vi "Webcam - Clamp Edges.vi"(0 "Image In":T1, 5 "Search Area Left":i32, 7 "Search Area Top":i32, 9 "Search Area Right":i32, 11 "Search Area Bottom":i32, 12 "Settings":T2={"Contrast"=100, "Filter width"=100, "Steepness"=2, "Subsampling Ratio"=1, "Show Search Area"=FALSE, "Show Search Lines"=FALSE, "Show Edges Found"=FALSE, "Show Result"=FALSE}) -> (4 "Image Out":T1, 6 "Left":sgl, 8 "Bottom":sgl, 10 "Right":sgl, 15 "Top":sgl)   [LabVIEW 2011]
uses:
  <vilib>/vision/Image Controls.llb/IMAQ Image.ctl
  <vilib>/vision/NI_Vision_Development_Module.lvlib
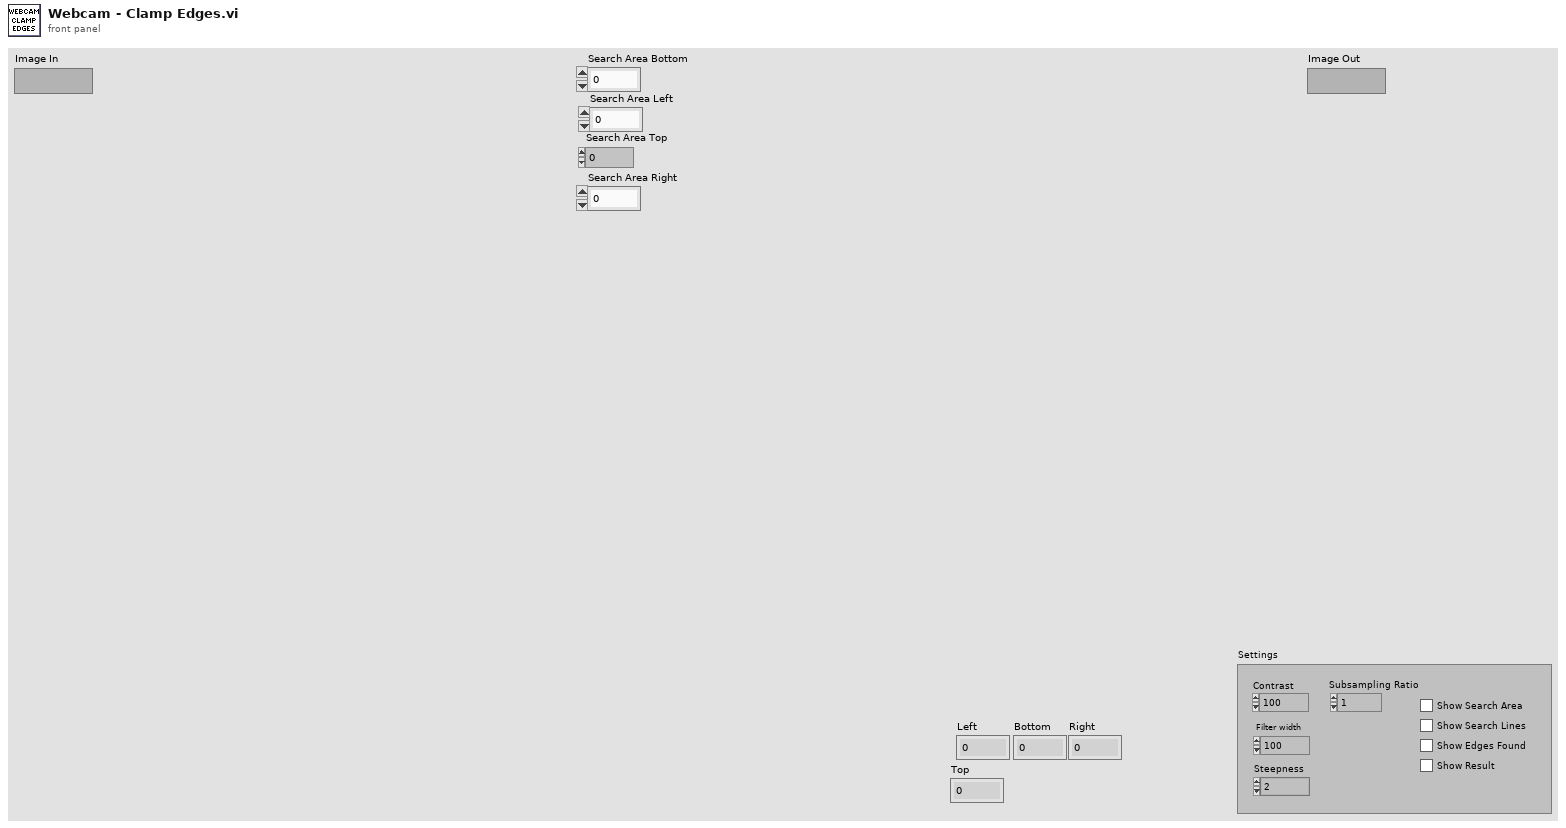
[diagram p1: front panel]
types:
  T1 = typedef "IMAQ Image.ctl" = refnum<image>
  T2 = cluster{"Contrast":i32, "Filter width":i32, "Steepness":i32, "Subsampling Ratio":u32, "Show Search Area":bool, "Show Search Lines":bool, "Show Edges Found":bool, "Show Result":bool}
  T3 = typedef "IMAQ Rectangle" = cluster{"Left":i32, "Top":i32, "Right":i32, "Bottom":i32, "Rotation":dbl}
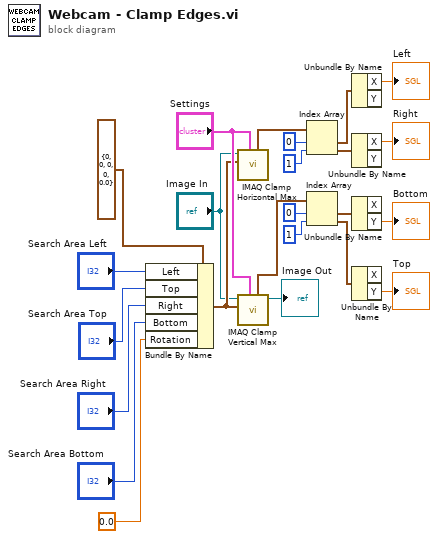
[diagram p0: block diagram]
diagram:
  n1 = Bundle By Name(cluster=T3 {"Left"=0, "Top"=0, "Right"=0, "Bottom"=0, "Rotation"=0.0} ("Rectangle"), "Left"="Search Area Left", "Top"="Search Area Top", "Right"="Search Area Right", "Bottom"="Search Area Bottom", "Rotation"=0.0) -> (w12:T3)
  n2 = call "IMAQ Clamp Horizontal Max"("Settings"="Settings", "Rectangle"=w12, "Image"="Image In") -> ("Edge Coordinates"=w20:cluster{"X":sgl, "Y":sgl}[])  [unwired: 4 in, 4 out]
  n3 = call "IMAQ Clamp Vertical Max"("Settings"="Settings", "Rectangle"=w12, "Image"="Image In") -> ("Image Out"=→"Image Out":T1, "Edge Coordinates"=w14:cluster{"X":sgl, "Y":sgl}[])  [unwired: 4 in, 3 out]
  n4 = Index Array(array=w20, index #1=0 ("index"), index #2=1 ("index")) -> (element #1=w23:cluster{"X":sgl, "Y":sgl}, element #2=w24:cluster{"X":sgl, "Y":sgl})
  n5 = Index Array(array=w14, index #1=0 ("index"), index #2=1 ("index")) -> (element #1=w16:cluster{"X":sgl, "Y":sgl}, element #2=w15:cluster{"X":sgl, "Y":sgl})
  n6 = Unbundle By Name(w23) -> ("X"=→"Left":sgl)  [unwired: 1 out]
  n7 = Unbundle By Name(w24) -> ("X"=→"Right":sgl)  [unwired: 1 out]
  n8 = Unbundle By Name(w16) -> ("Y"=→"Bottom":sgl)  [unwired: 1 out]
  n9 = Unbundle By Name(w15) -> ("Y"=→"Top":sgl)  [unwired: 1 out]
